vi "VariantToDBL.vi"(8 "error in":errorcluster, 11 "variant":variant) -> (0 "error out":errorcluster, 3 "data":dbl)   [LabVIEW 2017]
doc: "This VI converts <B>variant</B> to <B>DBL</B>. If none of the known data types or string is passed as variant, \"NaN\" is returned."
uses:
  <vilib>/Utility/Data Type/NI_Data Type.lvlib
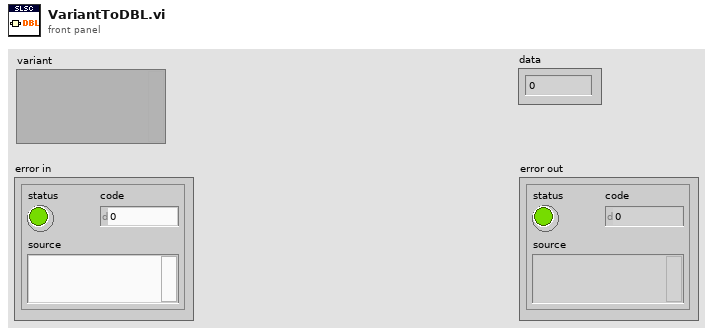
[diagram p1: front panel]
types:
  T1 = typedef "NI_Data Type.lvlib/Data Type.ctl" = enum8{"Invalid Type", "Void", "I8", "I16", "I32", "I64", "U8", "U16", "U32", "U64", "Single Float", "Double Float", "Extended Float", "Single Complex", "Double Complex", "Extended Complex", "Enum U8", "Enum U16", "Enum U32", "Enum U64", "Single Float With Unit", "Double Float With Unit", "Extended Float With Unit", "Single Complex with Unit", "Double Complex with Unit", "Extended Complex with Unit", "Boolean", "String", "Path", "Picture", "Tag", "Array", "Cluster", "Variant", "LV Variant", "Waveform", "Timestamp", "Digital Waveform", "Digital Data", "ExpressData", "Refnum", "External Data", "VI", "Poly VI", "LabVIEW Class Instance", "Fixed Point"}
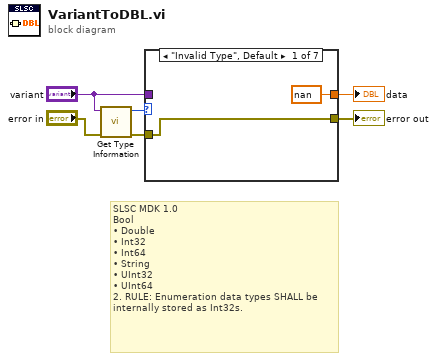
[diagram p0: block diagram]
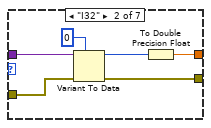
[diagram p2: hidden frame]
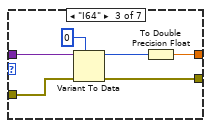
[diagram p3: hidden frame]
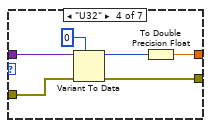
[diagram p4: hidden frame]
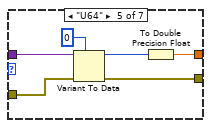
[diagram p5: hidden frame]
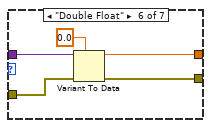
[diagram p6: hidden frame]
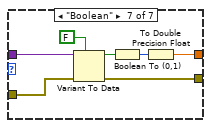
[diagram p7: hidden frame]
diagram:
  # "SLSC MDK 1.0 \nBool\n• Double\n• Int32\n• Int64\n• String\n• UInt32\n• UInt64\n2. RULE: Enumeration data types SHALL be\ninternally stored as Int32s."
  n1 = call <vilib>:"Get Type Information.vi"("error in (no error)"="error in", "Variant"="variant") -> ("error out"=w1:errorcluster, "Type"=w2:T1)  [unwired: 5 in, 3 out]
  n2 = case shown="\"Invalid Type\", Default" w2 {
    tunnel: w1 -> [w8 w14 w20 w26 w32 w37 w44]
    tunnel: "variant" -> [_ w13 w19 w25 w31 w36 w43]
    tunnel: [w8 w12 w18 w24 w30 w35 w42] -> w6
    tunnel: [nan w10 w16 w22 w28 w34 w40] -> w5
    frame "Invalid Type", Default {
    }
    frame "I32" {
      n3 = Variant To Data(error in=w14, type=0, Variant=w13) -> (data=w11:i32, error out=w12:errorcluster)
      n4 = To Double Precision Float(number=w11) -> (double precision float=w10:dbl)
    }
    frame "I64" {
      n5 = Variant To Data(error in=w20, type=i64 0, Variant=w19) -> (data=w17:i64, error out=w18:errorcluster)
      n6 = To Double Precision Float(number=w17) -> (double precision float=w16:dbl)
    }
    frame "U32" {
      n7 = Variant To Data(error in=w26, type=u32 0, Variant=w25) -> (data=w23:u32, error out=w24:errorcluster)
      n8 = To Double Precision Float(number=w23) -> (double precision float=w22:dbl)
    }
    frame "U64" {
      n9 = Variant To Data(error in=w32, type=u64 0, Variant=w31) -> (data=w29:u64, error out=w30:errorcluster)
      n10 = To Double Precision Float(number=w29) -> (double precision float=w28:dbl)
    }
    frame "Double Float" {
      n11 = Variant To Data(error in=w37, type=0.0, Variant=w36) -> (data=w34:dbl, error out=w35:errorcluster)
    }
    frame "Boolean" {
      n12 = Variant To Data(error in=w44, type=FALSE, Variant=w43) -> (data=w41:bool, error out=w42:errorcluster)
      n13 = Boolean To (0,1)(Boolean=w41) -> (0, 1=w38:i16)
      n14 = To Double Precision Float(number=w38) -> (double precision float=w40:dbl)
    }
  }
  "error out" <- w6
  "data" <- w5
